vi "GetNumericTextReference.vi"(8 "error in":errorcluster, 11 "Numeric Text in":refnum<class "NumericText.lvclass">) -> (0 "error out":errorcluster, 1 "NumericText reference":refnum<vi>, 3 "Numeric Text out":refnum<class "NumericText.lvclass">)   [LabVIEW 2014, in "NumericText.lvclass"]
uses:
  NumericText.lvclass
  Generic/Generic.lvclass
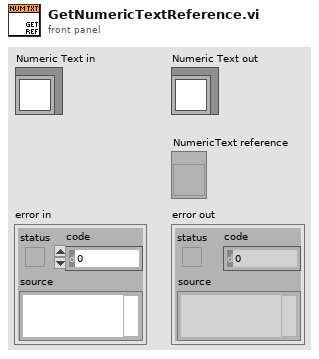
[diagram p1: front panel]
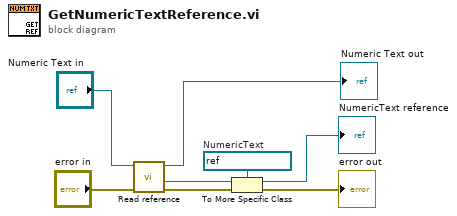
[diagram p0: block diagram]
diagram:
  w8 = refnum<vi> refnum  # NumericText
  n1 = call "Read reference.vi"("error in"="error in", "GObject in"="Numeric Text in") -> ("error out"=w3:errorcluster, "reference"=w2:refnum<vi>, "GObject out"=→"Numeric Text out":refnum<class "NumericText.lvclass">)  [unwired: 5 in]
  n2 = To More Specific Class(target class=w8, reference=w2, error in=w3) -> (specific class reference=→"NumericText reference":refnum<vi>, error out=→"error out":errorcluster)
